vi "Handle Messages.vi"(8 "error in (no error)":errorcluster, 9 "Message Data":variant, 10 "Message":string, 11 "Mock Rig Process In":refnum<class "Mock Process.lvclass">) -> (0 "error out":errorcluster, 3 "Mock Rig Process Out":refnum<class "Mock Process.lvclass">)   [LabVIEW 2020, in "Mock Process.lvclass"]
uses:
  Mock Process.lvclass
  Mock Process.lvclass/Mock Process.ctl
  Framework/Process/Process.lvclass
  Framework/Helper Loop/Helper Loop.lvclass
  C:/Git/triarc-framework/source/Framework/Process/Process.lvclass
  C:/Git/triarc-framework/source/Framework/Helper Loop/Helper Loop.lvclass
  <vilib>/ErrorRing/Error Ring.xnode
  <vilib>/Utility/error.llb/Error Cluster From Error Code.vi
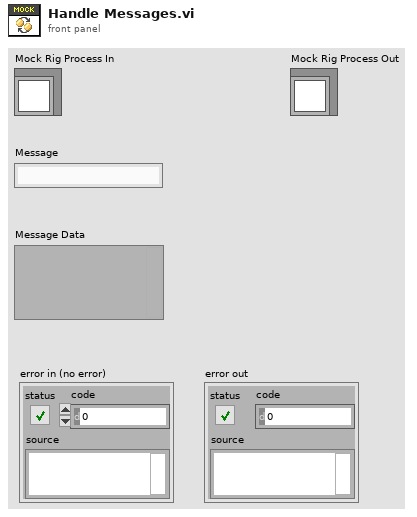
[diagram p1: front panel]
types:
  T1 = cluster{"Message":string, "Message Data":variant}
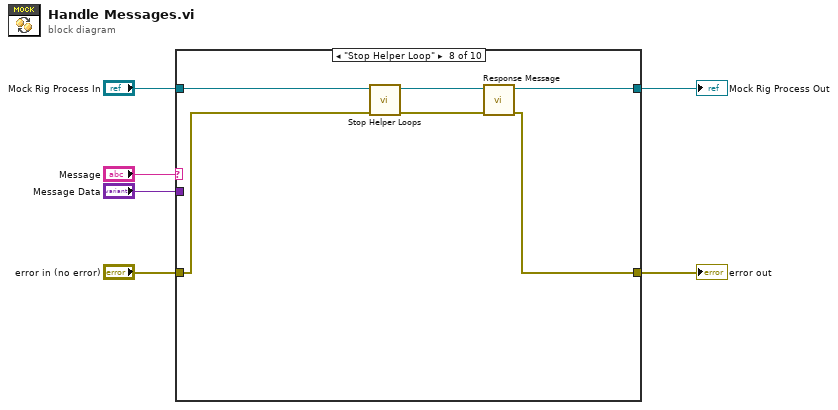
[diagram p0: block diagram]
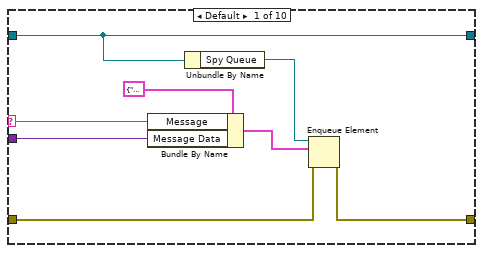
[diagram p2: hidden frame]
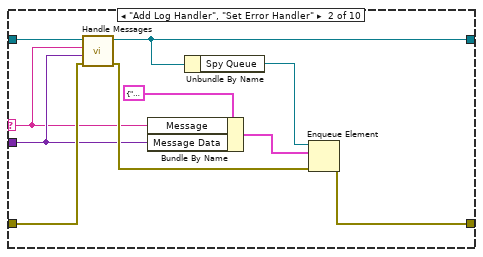
[diagram p3: hidden frame]
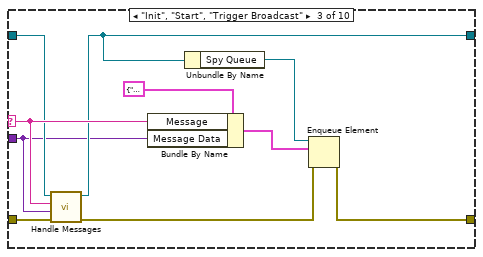
[diagram p4: hidden frame]
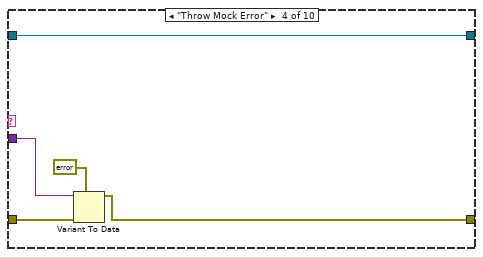
[diagram p5: hidden frame]
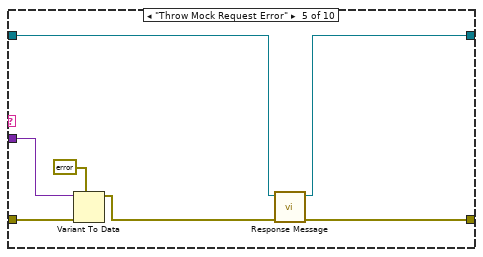
[diagram p6: hidden frame]
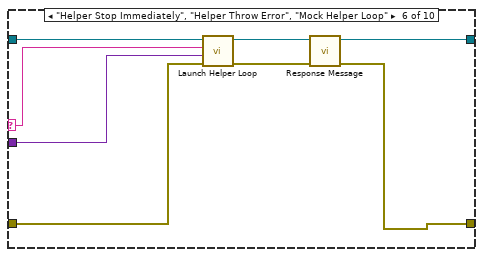
[diagram p7: hidden frame]
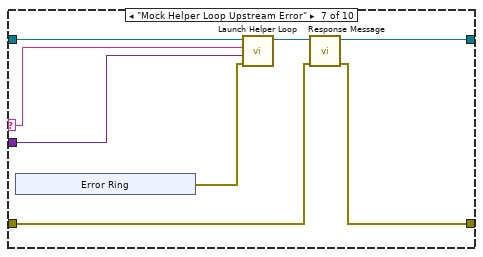
[diagram p8: hidden frame]
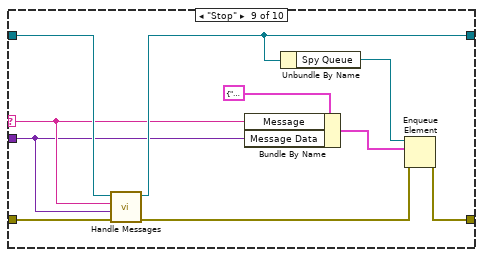
[diagram p9: hidden frame]
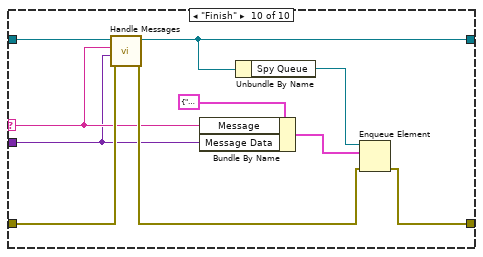
[diagram p10: hidden frame]
diagram:
  n1 = case shown="\"Stop Helper Loop\"" "Message" {
    selector: "Message" -> [w10 w15 w28 _ _ w51 w61 _ w74 w84]
    tunnel: [w8 w20 w30 w35 w42 w49 w59 w69 w79 w85] -> w6
    tunnel: [w7 w17 w27 w39 w41 w47 w57 w67 w76 w87] -> w5
    tunnel: "error in (no error)" -> [w9 w21 w31 w38 w46 w53 w56 w71 w77 w91]
    tunnel: "Message Data" -> [w11 w16 w25 w37 w45 w50 w60 _ w73 w83]
    tunnel: "Mock Rig Process In" -> [w7 w18 w26 w39 w40 w54 w62 w72 w75 w92]
    frame Default {
      n2 = Bundle By Name(cluster=T1 {"Message"="", "Message Data"=variant} ("Message Cluster"), "Message"=w10, "Message Data"=w11) -> (w14:T1)
      n3 = Unbundle By Name(w7) -> ("Spy Queue"=w12:refnum<queue>)
      n4 = Enqueue Element(queue=w12, element=w14, error in (no error)=w9) -> (error out=w8:errorcluster)  [unwired: 1 in, 2 out]
    }
    frame "Add Log Handler", "Set Error Handler" {
      n5 = call-parent "Handle Messages.vi"("error in (no error)"=w21, "Message Data"=w16, "Message"=w15, "Process In"=w18) -> ("error out"=w19:errorcluster, "Process Out"=w17:refnum<class "Mock Process.lvclass">)  [unwired: 6 in]
      n6 = Bundle By Name(cluster=T1 {"Message"="", "Message Data"=variant} ("Message Cluster"), "Message"=w15, "Message Data"=w16) -> (w24:T1)
      n7 = Unbundle By Name(w17) -> ("Spy Queue"=w22:refnum<queue>)
      n8 = Enqueue Element(queue=w22, element=w24, error in (no error)=w19) -> (error out=w20:errorcluster)  [unwired: 1 in, 2 out]
    }
    frame "Init", "Start", "Trigger Broadcast" {
      n9 = call-parent "Handle Messages.vi"("error in (no error)"=w31, "Message Data"=w25, "Message"=w28, "Process In"=w26) -> ("error out"=w29:errorcluster, "Process Out"=w27:refnum<class "Mock Process.lvclass">)  [unwired: 6 in]
      n10 = Bundle By Name(cluster=T1 {"Message"="", "Message Data"=variant} ("Message Cluster"), "Message"=w28, "Message Data"=w25) -> (w34:T1)
      n11 = Unbundle By Name(w27) -> ("Spy Queue"=w32:refnum<queue>)
      n12 = Enqueue Element(queue=w32, element=w34, error in (no error)=w29) -> (error out=w30:errorcluster)  [unwired: 1 in, 2 out]
    }
    frame "Throw Mock Error" {
      n13 = Variant To Data(error in=w38, type=errorcluster {"status"=FALSE, "code"=0, "source"=""} ("error out"), Variant=w37) -> (data=w35:errorcluster)  [unwired: 1 out]
    }
    frame "Throw Mock Request Error" {
      n14 = Variant To Data(error in=w46, type=errorcluster {"status"=FALSE, "code"=0, "source"=""} ("error out"), Variant=w45) -> (data=w43:errorcluster)  [unwired: 1 out]
      n15 = call "Response Message.vi"("error in (no error)"=w43, "Process In"=w40) -> ("error out"=w42:errorcluster, "Process Out"=w41:refnum<class "Mock Process.lvclass">)  [unwired: 8 in]
    }
    frame "Helper Stop Immediately", "Helper Throw Error", "Mock Helper Loop" {
      n16 = call "Launch Helper Loop.vi"("error in (no error)"=w53, "Message Data"=w50, "Message"=w51, "Helper Loop In"=w54) -> ("error out"=w52:errorcluster, "Helper Loop Out"=w48:refnum<class "Mock Process.lvclass">)  [unwired: 6 in]
      n17 = call "Response Message.vi"("error in (no error)"=w52, "Process In"=w48) -> ("error out"=w49:errorcluster, "Process Out"=w47:refnum<class "Mock Process.lvclass">)  [unwired: 8 in]
    }
    frame "Mock Helper Loop Upstream Error" {
      n18 = xnode "Error Ring"() -> ("error out"=w55:errorcluster)
      n19 = call "Launch Helper Loop.vi"("error in (no error)"=w55, "Message Data"=w60, "Message"=w61, "Helper Loop In"=w62) -> ("Helper Loop Out"=w58:refnum<class "Mock Process.lvclass">)  [unwired: 6 in, 1 out]
      n20 = call "Response Message.vi"("error in (no error)"=w56, "Process In"=w58) -> ("error out"=w59:errorcluster, "Process Out"=w57:refnum<class "Mock Process.lvclass">)  [unwired: 8 in]
    }
    frame "Stop Helper Loop" {
      n21 = call "Stop Helper Loops.vi"("error in (no error)"=w71, "Helper Loop In"=w72) -> ("error out"=w70:errorcluster, "Helper Loop Out"=w68:refnum<class "Mock Process.lvclass">)  [unwired: 8 in]
      n22 = call "Response Message.vi"("error in (no error)"=w70, "Process In"=w68) -> ("error out"=w69:errorcluster, "Process Out"=w67:refnum<class "Mock Process.lvclass">)  [unwired: 8 in]
    }
    frame "Stop" {
      n23 = call-parent "Handle Messages.vi"("error in (no error)"=w77, "Message Data"=w73, "Message"=w74, "Process In"=w75) -> ("error out"=w78:errorcluster, "Process Out"=w76:refnum<class "Mock Process.lvclass">)  [unwired: 6 in]
      n24 = Bundle By Name(cluster=T1 {"Message"="", "Message Data"=variant} ("Message Cluster"), "Message"=w74, "Message Data"=w73) -> (w82:T1)
      n25 = Unbundle By Name(w76) -> ("Spy Queue"=w80:refnum<queue>)
      n26 = Enqueue Element(queue=w80, element=w82, error in (no error)=w78) -> (error out=w79:errorcluster)  [unwired: 1 in, 2 out]
    }
    frame "Finish" {
      n27 = call-parent "Handle Messages.vi"("error in (no error)"=w91, "Message Data"=w83, "Message"=w84, "Process In"=w92) -> ("error out"=w86:errorcluster, "Process Out"=w87:refnum<class "Mock Process.lvclass">)  [unwired: 6 in]
      n28 = Bundle By Name(cluster=T1 {"Message"="", "Message Data"=variant} ("Message Cluster"), "Message"=w84, "Message Data"=w83) -> (w90:T1)
      n29 = Unbundle By Name(w87) -> ("Spy Queue"=w89:refnum<queue>)
      n30 = Enqueue Element(queue=w89, element=w90, error in (no error)=w86) -> (error out=w85:errorcluster)  [unwired: 1 in, 2 out]
    }
  }
  "error out" <- w6
  "Mock Rig Process Out" <- w5
